vi "Agilent PWM Serial Connection.vi"(1 "VISA Resource Name":refnum<visa-resource-name>) -> (0 "Serial?":bool)   [LabVIEW 2011]
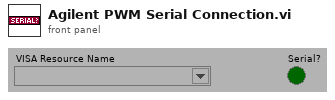
[diagram p1: front panel]
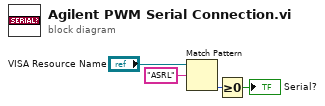
[diagram p0: block diagram]
diagram:
  n1 = Match Pattern(string="VISA Resource Name", regular expression="ASRL") -> (offset past match=w3:i32)  [unwired: 4 out]
  n2 = Greater Or Equal To 0?(x=w3) -> (x >= 0?=→"Serial?":bool)
